vi "Verify Array of Integers.vi"(8 "error in (no error)":errorcluster) -> (0 "error out":errorcluster)   [LabVIEW 2020]
uses:
  <vilib>/SAS/Approval Tests/Approval Tests/Options/Options.lvclass/Options.ctl
  <vilib>/SAS/Approval Tests/Approval Tests/Naming Data/Naming Data.lvclass/Naming Data.ctl
  <vilib>/SAS/Approval Tests/Approval Tests/Options/Options.lvclass
  <vilib>/SAS/Approval Tests/Approval Tests/Scrubber/Scrubber.lvclass
  <vilib>/SAS/Approval Tests/Approval Tests/Namer/Namer.lvclass
  <vilib>/SAS/Approval Tests/Approval Tests/Naming Data/Naming Data.lvclass
  <vilib>/SAS/Approval Tests/Approval Tests/Reporter/Reporter.lvclass
  <vilib>/SAS/Approval Tests/Approval Tests/Text Comparator/Text Comparator.lvclass
  a3cea956-c44a-453c-97a3-d1e04fce9a5d.vi
  <vilib>/addons/_JKI Toolkits/Caraya/classes/Test/Test.lvclass
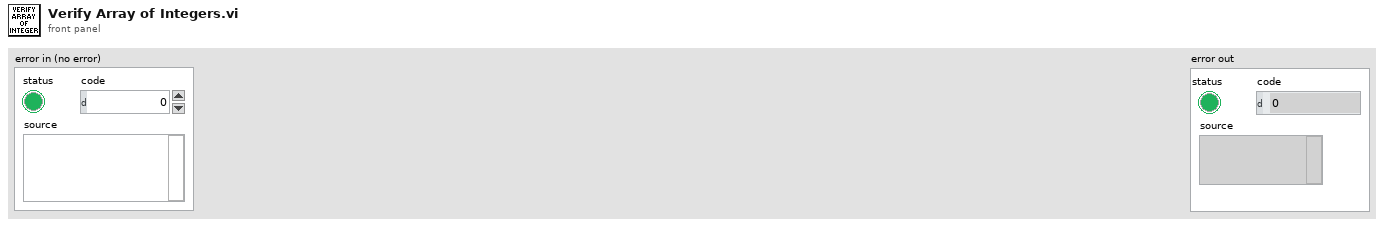
[diagram p1: front panel]
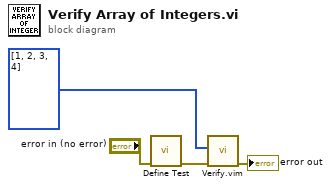
[diagram p0: block diagram]
diagram:
  n1 = call <vilib>:"Define Test.vi"("error in (no error)"="error in (no error)") -> ("error out"=w4:errorcluster)  [unwired: 9 in, 1 out]
  n2 = call "Verify.vim"("error in"=w4, "Test Data"=i32[] [1, 2, 3, 4]) -> ("error out"=→"error out":errorcluster)  [unwired: 8 in, 1 out]
